vi "RubikTurnFSM.vi"(1 "Turn":T3=enum."ccw", 2 "Servo Enum":T1) -> (0 "Turn State (out)":T2=enum."-90°")   [LabVIEW 2017]
uses:
  Projekt-RubikLibrary/ServoCCWControl.ctl
  Projekt-RubikLibrary/ServoAbsAngleControl.ctl
  Projekt-RubikLibrary/ServoEnumControl.ctl
  Projekt-RubikLibrary/RubikLibrary.lvlib
  Projekt-RubikLibrary/RubikLibraryRT.lvlib
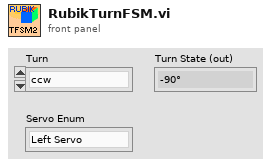
[diagram p1: front panel]
types:
  T1 = typedef "RubikLibrary.lvlib/ServoEnumControl.ctl" = enum16{"Left Servo", "Front Servo", "Right Servo"}
  T2 = typedef "RubikLibrary.lvlib/ServoAbsAngleControl.ctl" = enum16{"+90°", "0°", "-90°"}
  T3 = typedef "RubikLibrary.lvlib/ServoCCWControl.ctl" = enum16{"cw", "ccw"}
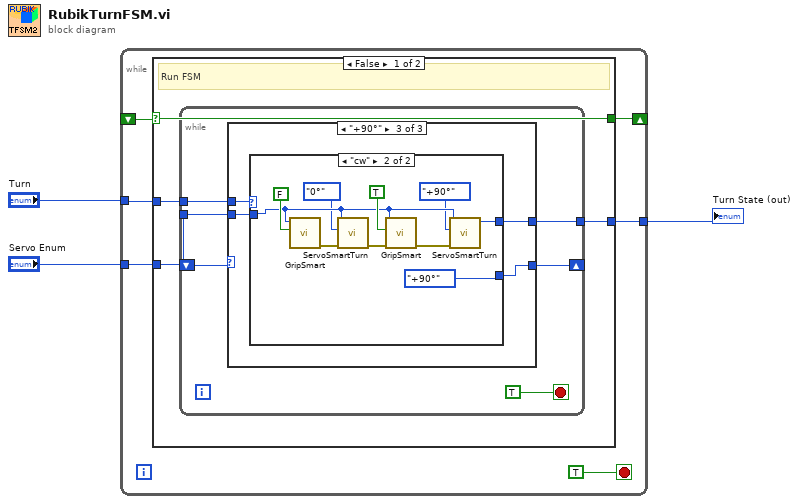
[diagram p0: block diagram]
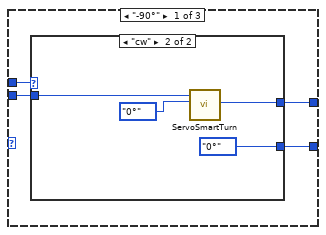
[diagram p2: hidden frame]
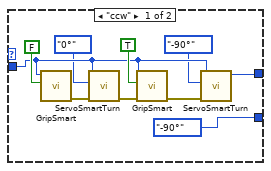
[diagram p3: hidden frame]
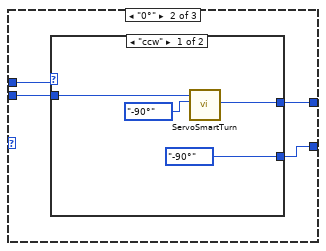
[diagram p4: hidden frame]
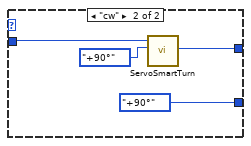
[diagram p5: hidden frame]
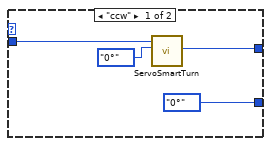
[diagram p6: hidden frame]
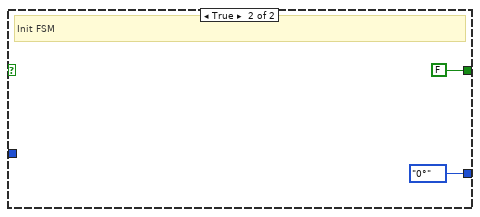
[diagram p7: hidden frame]
diagram:
  n1 = while {
    tunnel: "Turn" -> [w9]
    tunnel: [w8] -> w2
    tunnel: "Servo Enum" -> [w7]
    shift-right: [w4] -> _
    shift-left: _ -> [w5]
    stop <- TRUE stop-if-true
    n2 = case shown="False" w5 {
      selector: w5 -> [w10 _]
      tunnel: w9 -> [w13 _]
      tunnel: [w12 ServoAbsAngleControl."0°" ("Turn State (out)")] -> w8
      tunnel: w7 -> [w11 _]
      tunnel: [w10 FALSE] -> w4
      frame False {
        # "Run FSM"
        n3 = while {
          shift-right: [w18] -> _
          shift-left: _ -> [w19]
          tunnel: w11 -> [w16]
          tunnel: [w15] -> w12
          tunnel: w13 -> [w14]
          stop <- TRUE stop-if-true
          n4 = case shown="\"+90°\"" w19 {
            tunnel: [w23 w41 w53] -> w18
            tunnel: w16 -> [w22 w40 w52]
            tunnel: [w21 w39 w51] -> w15
            tunnel: w14 -> [w20 w38 w50]
            frame "-90°" {
              n5 = case shown="\"cw\"" w20 {
                tunnel: [ServoAbsAngleControl."-90°" ("Enum 2") ServoAbsAngleControl."0°" ("Enum 2")] -> w23
                tunnel: w22 -> [w27 w36]
                tunnel: [w26 w35] -> w21
                frame "ccw" {
                  n6 = call "GripSmart.vi"("Grip closed (in)"=FALSE ("Turn to (in)"), "Servo"=w27) -> ("error out"=w31:errorcluster)  [unwired: 8 in, 1 out]
                  n7 = call "ServoSmartTurn.vi"("error in"=w31, "Turn to (in)"=ServoAbsAngleControl."0°" ("Turn to"), "Servo"=w27) -> ("error out"=w30:errorcluster)  [unwired: 7 in, 1 out]
                  n8 = call "GripSmart.vi"("error in"=w30, "Grip closed (in)"=TRUE ("Turn to (in)"), "Servo"=w27) -> ("error out"=w29:errorcluster)  [unwired: 7 in, 1 out]
                  n9 = call "ServoSmartTurn.vi"("error in"=w29, "Turn to (in)"=ServoAbsAngleControl."-90°" ("Turn to"), "Servo"=w27) -> ("Turn State (out)"=w26:T2)  [unwired: 7 in, 1 out]
                }
                frame "cw" {
                  n10 = call "ServoSmartTurn.vi"("Turn to (in)"=ServoAbsAngleControl."0°" ("Turn to"), "Servo"=w36) -> ("Turn State (out)"=w35:T2)  [unwired: 8 in, 1 out]
                }
              }
            }
            frame "0°" {
              n11 = case shown="\"ccw\"" w38 {
                tunnel: [ServoAbsAngleControl."-90°" ("Enum 2") ServoAbsAngleControl."+90°" ("Enum 2")] -> w41
                tunnel: w40 -> [w44 w48]
                tunnel: [w43 w47] -> w39
                frame "ccw" {
                  n12 = call "ServoSmartTurn.vi"("Turn to (in)"=ServoAbsAngleControl."-90°" ("Turn to"), "Servo"=w44) -> ("Turn State (out)"=w43:T2)  [unwired: 8 in, 1 out]
                }
                frame "cw" {
                  n13 = call "ServoSmartTurn.vi"("Turn to (in)"=ServoAbsAngleControl."+90°" ("Turn to"), "Servo"=w48) -> ("Turn State (out)"=w47:T2)  [unwired: 8 in, 1 out]
                }
              }
            }
            frame "+90°" {
              n14 = case shown="\"cw\"" w50 {
                tunnel: [ServoAbsAngleControl."0°" ("Enum 2") ServoAbsAngleControl."+90°" ("Enum 2")] -> w53
                tunnel: w52 -> [w56 w61]
                tunnel: [w55 w60] -> w51
                frame "ccw" {
                  n15 = call "ServoSmartTurn.vi"("Turn to (in)"=ServoAbsAngleControl."0°" ("Turn to"), "Servo"=w56) -> ("Turn State (out)"=w55:T2)  [unwired: 8 in, 1 out]
                }
                frame "cw" {
                  n16 = call "GripSmart.vi"("Grip closed (in)"=FALSE ("Turn to (in)"), "Servo"=w61) -> ("error out"=w65:errorcluster)  [unwired: 8 in, 1 out]
                  n17 = call "ServoSmartTurn.vi"("error in"=w65, "Turn to (in)"=ServoAbsAngleControl."0°" ("Turn to"), "Servo"=w61) -> ("error out"=w64:errorcluster)  [unwired: 7 in, 1 out]
                  n18 = call "GripSmart.vi"("error in"=w64, "Grip closed (in)"=TRUE ("Turn to (in)"), "Servo"=w61) -> ("error out"=w63:errorcluster)  [unwired: 7 in, 1 out]
                  n19 = call "ServoSmartTurn.vi"("error in"=w63, "Turn to (in)"=ServoAbsAngleControl."+90°" ("Turn to"), "Servo"=w61) -> ("Turn State (out)"=w60:T2)  [unwired: 7 in, 1 out]
                }
              }
            }
          }
        }
      }
      frame True {
        # "Init FSM"
      }
    }
  }
  "Turn State (out)" <- w2
